vi "Write Data_Test Firebase.vi"(8 "error in (no error)":errorcluster caption="entrée d'erreur (pas d'erreur)", 11 "Actor Test Firebase en entrée":refnum<class "Actor Test Firebase.lvclass">) -> (0 "error out":errorcluster caption="sortie d'erreur", 3 "Actor Test Firebase en sortie":refnum<class "Actor Test Firebase.lvclass">)   [LabVIEW 2020, in "Library Core.lvlib" / "Actor Test Firebase.lvclass"]
uses:
  Actor Test Firebase.lvclass
  C:/Users/ngarcin/OneDrive - Altyor/Standard TB/Class/Sequencer/Actor Test (Default)/Actor Test (Default).lvclass
  Commun VI/TypeDef/Commande Test/Commande Value Type.ctl
  Commun VI/TypeDef/Command firebase altyor/Parameter Firebase Altyor.ctl
  Commun VI/TypeDef/Bench Type.ctl
  Firebase/Source/Firebase Altyor/Firebase Altyor.lvclass
  Commun VI/TypeDef/Liste Error.ctl
  JSON API/JSON Value/Set from JSON string.vi
  JSON API/Variant JSON/Variant to JSON.vi
  JSON API/JSON Value/Get Item by name array.vi
  Sequencer (Default)/Sequencer (Default).lvclass
  Instrument/Instrument (Default)/Class Instrument (Default).lvclass
  JSON API/JSON Value/JSON Value.lvclass
  Actor Test Firebase.lvclass/Actor Test Firebase.ctl
  JSON API/Variant JSON/Variant JSON.lvlib
  JSON API/Get Polymorphic/JSON GetSet.lvlib
  Commun VI/Library Commun.lvlib
panel:
  in  "TypeValue":T1
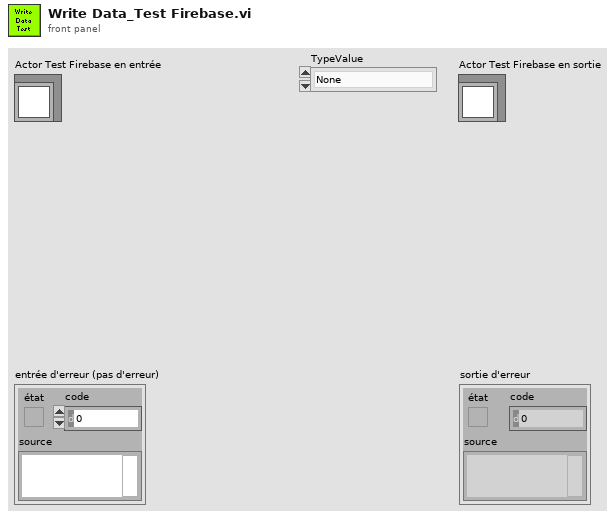
[diagram p1: front panel]
types:
  T1 = typedef "Library Commun.lvlib/Commande Value Type.ctl" = enum16{"None", "String", "Number", "Timestamp", "Boolean", "Array"}
  T2 = typedef "Library Commun.lvlib/Liste Error.ctl" = enum16{"Firebase Driver - Get Document", "Firebase Driver - Get Document With Where", "Firebase Driver - Delete Document", "Firebase Driver - Set Document", "Firebase Driver - Update Document", "Firebase Altyor - Search Document Bench", "Firebase Altyor - Class Not in Firebase", "Spectrum_Analyser - Timeout", "Relay Board - Qty Relay", "DIO - Pb Funtion", "Power_Supply - Peripherical not find", "Mutimeter - Peripherical not find", "Instrument - Function Not Used", "Instrument - Instrument name not specified", "Instrument - Allready Initialised", "Instrument - TimeOut", "Instrument - the instrument must be Initialise before", "Instrument - Frame Not received", "Instrument - Frame Nok", "Test - Initialise the File_for_Save", "Test - Timeout", "Test - Cmd Error", "FGV - Variable ", "BDD FireBase - Define Class", "SN - Class Not Define"}
  T3 = typedef "Library Commun.lvlib/Bench Type.ctl" = enum16{"Bench PCBA", "Bench Camera", "Bench Assembly", "Bench PCBA P2193"}
  T4 = typedef "Library Commun.lvlib/Parameter Firebase Altyor.ctl" = cluster{"Name_BDD":string, "API_Key":string, "Nb_to_Read":string, "Value_to_find":string, "Field_Filter":string, "Field_Order":string, "Collection_to_find":string, "Name_Bench":string, "Bench Type":T3, "Type Data ":enum16{"Data Product", "Data Test"}, "Firebase Altyor":refnum<class "Firebase Altyor.lvclass">}
  T5 = typedef "Library Commun.lvlib/Commande Type Test.ctl" = enum16{"Function", "Test", "Calculation"}
  T6 = cluster{"Main Test":string, "Name Test":string, "StartOfTest":string, "Value":string, "Limit_Low":string, "Limit_High":string, "Result":bool, "Fatal_Test":bool, "NbRetry":dbl, "EndOfTest":string, "Error":string, "TypeValue":T1, "Type Test":T5}[]
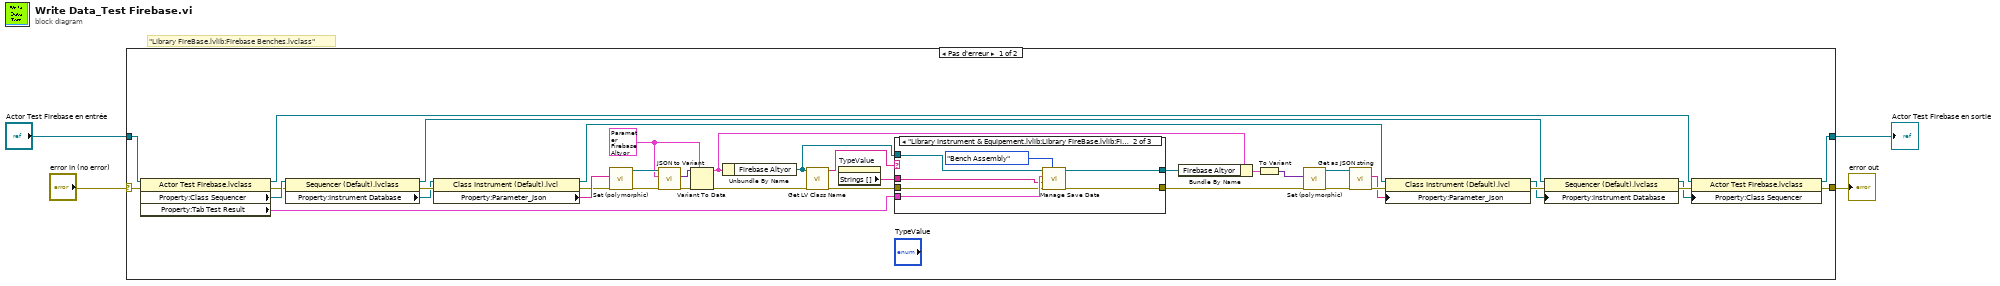
[diagram p0: block diagram]
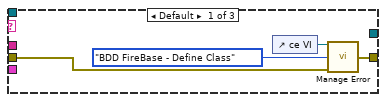
[diagram p2: hidden frame]
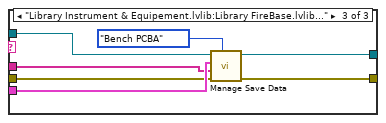
[diagram p3: hidden frame]
diagram:
  # "\"Library FireBase.lvlib:Firebase Benches.lvclass\""
  n1 = case shown="Pas d'erreur" "error in (no error)" {
    selector: "error in (no error)" -> [w39 w60]
    tunnel: [w6 w61] -> w2
    tunnel: "Actor Test Firebase en entrée" -> [w40 w61]
    tunnel: [w9 w60] -> w1
    frame No Error {
      w5 = T4 {"Name_BDD"="", "API_Key"="", "Nb_to_Read"="", "Value_to_find"="", "Field_Filter"="", "Field_Order"="", "Collection_to_find"="", "Name_Bench"="", "Bench Type"=enum."Bench PCBA", "Type Data "=enum."Data Product", "Firebase Altyor"=refnum} ("Parameter")
      n2 = property class="Actor Test Firebase.lvclass"(reference=w40, error in=w39) -> (reference out=w10:refnum<class "Actor Test Firebase.lvclass">, error out=w38:errorcluster, "Property:Class Sequencer"=w41:refnum<class "Sequencer (Default).lvclass">, "Property:Tab Test Result"=w25:T6)
      n3 = property class="Sequencer (Default).lvclass"(reference=w41, error in=w38) -> (reference out=w13:refnum<class "Sequencer (Default).lvclass">, error out=w30:errorcluster, "Property:Instrument Database"=w29:refnum<class "Class Instrument (Default).lvclass">)
      n4 = property class="Class Instrument (Default).lvcl"(reference=w29, error in=w30) -> (reference out=w14:refnum<class "Class Instrument (Default).lvclass">, error out=w31:errorcluster, "Property:Parameter_Json"=w33:string)
      n5 = call-poly "Set (polymorphic).vi"("error in (no error)"=w31, "JSON stream"=w33) -> ("error out"=w35:errorcluster, "JSON Value out"=w37:refnum<class "JSON Value.lvclass">)  [unwired: 7 in, 1 out]
      n6 = call "JSON to Variant.vi"("error in (no error)"=w35, "Variant (Data Type)"=w5, "JSON Value"=w37) -> ("error out"=w36:errorcluster, "Variant out"=w34:variant)  [unwired: 7 in]
      n7 = Variant To Data(error in=w36, type=w5, Variant=w34) -> (data=w7:T4, error out=w32:errorcluster)
      n8 = Unbundle By Name(w7) -> ("Firebase Altyor"=w26:refnum<class "Firebase Altyor.lvclass">)
      n9 = call <vilib>:"Get LV Class Name.vi"("error in (no error)"=w32, "object"=w26) -> ("error out"=w27:errorcluster, "class name"=w28:string)  [unwired: 8 in]
      n10 = property on="TypeValue" class="Énum (strict)"() -> ("Strings []"=w8:string[])  [unwired: 2 in, 2 out]
      n11 = case shown="\"Library Instrument & Equipement.lvlib:Library FireBase.lvlib:Firebase AssembledProducts.lvclass\"" w28 {
        tunnel: [w43 w52 w59] -> w15
        tunnel: w27 -> [w42 w48 w55]
        tunnel: w26 -> [_ w47 w54]
        tunnel: w25 -> [_ w51 w58]
        tunnel: [_ w50 w57] -> w16
        tunnel: w8 -> [_ w49 w56]
        frame Default {
          n12 = control-ref of="ce VI"() -> (w44:refnum<vi>)
          n13 = call "Manage Error.vi"("VI in Error"=w44, "Code Erreur"=Liste_Error."BDD FireBase - Define Class", "error in (no error)"=w42) -> ("error out"=w43:errorcluster)  [unwired: 12 in]
        }
        frame "Library Instrument & Equipement.lvlib:Library FireBase.lvlib:Firebase AssembledProducts.lvclass" {
          n14 = call "Manage Save Data.vi"("Bench Type"=Bench_Type."Bench Assembly", "entrée d'erreur (pas d'erreur)"=w48, "Strings []"=w49, "Property:Tab Test Result"=w51, "Firebase Altyor en entrée"=w47) -> ("sortie d'erreur"=w52:errorcluster, "Firebase Altyor en sortie"=w50:refnum<class "Firebase Altyor.lvclass">)  [unwired: 5 in]
        }
        frame "Library Instrument & Equipement.lvlib:Library FireBase.lvlib:Firebase Benches.lvclass" {
          n15 = call "Manage Save Data.vi"("Bench Type"=Bench_Type."Bench PCBA", "entrée d'erreur (pas d'erreur)"=w55, "Strings []"=w56, "Property:Tab Test Result"=w58, "Firebase Altyor en entrée"=w54) -> ("sortie d'erreur"=w59:errorcluster, "Firebase Altyor en sortie"=w57:refnum<class "Firebase Altyor.lvclass">)  [unwired: 5 in]
        }
      }
      n16 = Bundle By Name(cluster=w7, "Firebase Altyor"=w16) -> (w20:T4)
      n17 = To Variant(anything=w20) -> (Variant=w17:variant)
      n18 = call-poly "Set (polymorphic).vi"("error in (no error)"=w15, "Variant"=w17) -> ("error out"=w19:errorcluster, "JSON Value out"=w18:refnum<class "JSON Value.lvclass">)  [unwired: 8 in]
      n19 = call "Get as JSON string.vi"("error in (no error)"=w19, "JSON Value in"=w18) -> ("error out"=w22:errorcluster, "<JSON>"=w21:string)  [unwired: 8 in]
      n20 = property class="Class Instrument (Default).lvcl"(reference=w14, error in=w22, "Property:Parameter_Json"=w21) -> (reference out=w23:refnum<class "Class Instrument (Default).lvclass">, error out=w24:errorcluster)
      n21 = property class="Sequencer (Default).lvclass"(reference=w13, error in=w24, "Property:Instrument Database"=w23) -> (reference out=w11:refnum<class "Sequencer (Default).lvclass">, error out=w12:errorcluster)
      n22 = property class="Actor Test Firebase.lvclass"(reference=w10, error in=w12, "Property:Class Sequencer"=w11) -> (reference out=w6:refnum<class "Actor Test Firebase.lvclass">, error out=w9:errorcluster)
    }
    frame Error {
    }
  }
  "error out" <- w1
  "Actor Test Firebase en sortie" <- w2
